vi "SDO_TRAJECTORY_EXECUTE_ABS.vi"(8 "Init":bool, 11 "End Pose ENG":T1={"TRANSLATION"={"X"=0.0, "Y"=0.0}, "ROTATION"={"VALUE"=0.0, "COS"=1.0, "SIN"=0.0}} {"ROTATION"."SIN" format="%13.4f"; "ROTATION"."COS" format="%13.4f"; "ROTATION"."VALUE" format="%13.4f"; "TRANSLATION"."Y" format="%14.3f"; "TRANSLATION"."X" format="%14.3f"}) -> (0 "AtReference":bool, 3 "Chassis Velocity Target":T4 {"vOmega" format="%10.3f"; "vY" format="%10.3f"; "vX" format="%10.3f"})   [LabVIEW 2023]
uses:
  <vilib>/Rock Robotics/WPI/ThirdParty/JAS_Junk/TrajLib/Trajectory_Library.lvlib
  SDO_TRAJECTORY_GLOBALS.vi
  <vilib>/Rock Robotics/WPI/ThirdParty/JAS_Junk/TrajLib/TypeDef/CHASSIS_SPEEDS.ctl
  <vilib>/Rock Robotics/WPI/ThirdParty/JAS_Junk/TrajLib/TypeDef/TRANSLATION2D.ctl
  <vilib>/Rock Robotics/WPI/ThirdParty/JAS_Junk/TrajLib/TypeDef/ROTATION2D.ctl
  <vilib>/Rock Robotics/WPI/ThirdParty/JAS_Junk/TrajLib/TypeDef/POSE2D.ctl
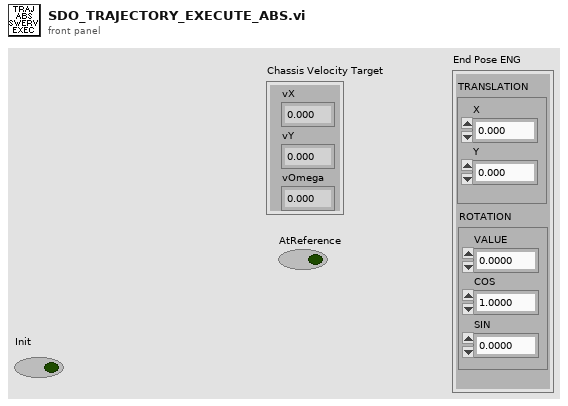
[diagram p1: front panel]
types:
  T1 = typedef "Trajectory_Library.lvlib/POSE2D.ctl" = cluster{"TRANSLATION":T2, "ROTATION":T3}
  T2 = typedef "Trajectory_Library.lvlib/TRANSLATION2D.ctl" = cluster{"X":dbl, "Y":dbl}
  T3 = typedef "Trajectory_Library.lvlib/ROTATION2D.ctl" = cluster{"VALUE":dbl, "COS":dbl, "SIN":dbl}
  T4 = typedef "Trajectory_Library.lvlib/CHASSIS_SPEEDS.ctl" = cluster{"vX":dbl, "vY":dbl, "vOmega":dbl}
  T5 = typedef "Trajectory_Library.lvlib/SWERVE_DRIVE_KINEMATICS.ctl" = cluster{"NumModules":i32, "InverseKinematics":T6, "ForwardKinematics":T6, "Modules":T2[], "PrevCoR":T2, "SavedModuleStates":T7[]}
  T6 = typedef "NI_Matrix.lvlib/RealMatrix.ctl" = dbl[][]
  T7 = typedef "Trajectory_Library.lvlib/SWERVE_DRIVE_MODULE_STATE.ctl" = cluster{"Speed":dbl, "Angle":T3}
  T8 = typedef "Trajectory_Library.lvlib/TRAJECTORY.ctl" = cluster{"TotalTImeSecs":dbl, "States":T9[]}
  T9 = typedef "Trajectory_Library.lvlib/TRAJ_STATE.ctl" = cluster{"TimeSeconds":dbl, "Velocity":dbl, "Acceleration":dbl, "POSE":T1, "Curvature":dbl}
  T10 = typedef "Trajectory_Library.lvlib/PID_TUNING.ctl" = cluster{"Kp":dbl, "Ki":dbl, "Kd":dbl, "MaximumIntegral":dbl, "MinimumIntegral":dbl}
  T11 = typedef "Trajectory_Library.lvlib/PROFILED_PID_CONTROLLER.ctl" = cluster{"Controller":T12, "Goal":T13, "Setpoint":T13, "Constraint":T14}
  T12 = typedef "Trajectory_Library.lvlib/PID_CONTROLLER.ctl" = cluster{"Kp":dbl, "Ki":dbl, "Kd":dbl, "Period":dbl, "Max_Integral":dbl, "Min_Integral":dbl, "Max_Input":dbl, "Min_Input":dbl, "Continuous":bool, "PositionError":dbl, "VelocityError":dbl, "PrevError":dbl, "TotalError":dbl, "PositionTolerance":dbl, "VelocityTolerance":dbl, "SetPoint":dbl, "Kf":dbl, "Prev_Deriv":dbl, "Prev_Deriv 2":dbl, "DerivativeFilter":bool, "Min_Output":dbl, "Max_Output":dbl, "Prev_F_P":dbl, "Prev_F_P_2":dbl, "AntiWindupActive":bool, "Measurement":dbl}
  T13 = typedef "Trajectory_Library.lvlib/TRAPEZOID_PROFILE_STATE.ctl" = cluster{"Position":dbl, "Velocity":dbl}
  T14 = typedef "Trajectory_Library.lvlib/TRAPEZOID_PROFILE_CONSTRAINT.ctl" = cluster{"MaxVelocity":dbl, "MaxAcceleration":dbl}
  T15 = typedef "Trajectory_Library.lvlib/HOLONOMIC_PACK_TUNING.ctl" = cluster{"X PID Tuning":T10, "Y PID Tuning":T10, "thetaProfiledPID_CTRL":T11}
  T16 = typedef "Trajectory_Library.lvlib/HOLONOMIC_DRV_CTRL.ctl" = cluster{"poseTolerance":T1, "poseError":T1, "Enabled":bool, "PID_xCtrl":T12, "PID_yCtrl":T12, "PROF_PID_thetaCtrl":T11, "RotationError":T3, "FirstRun":bool}
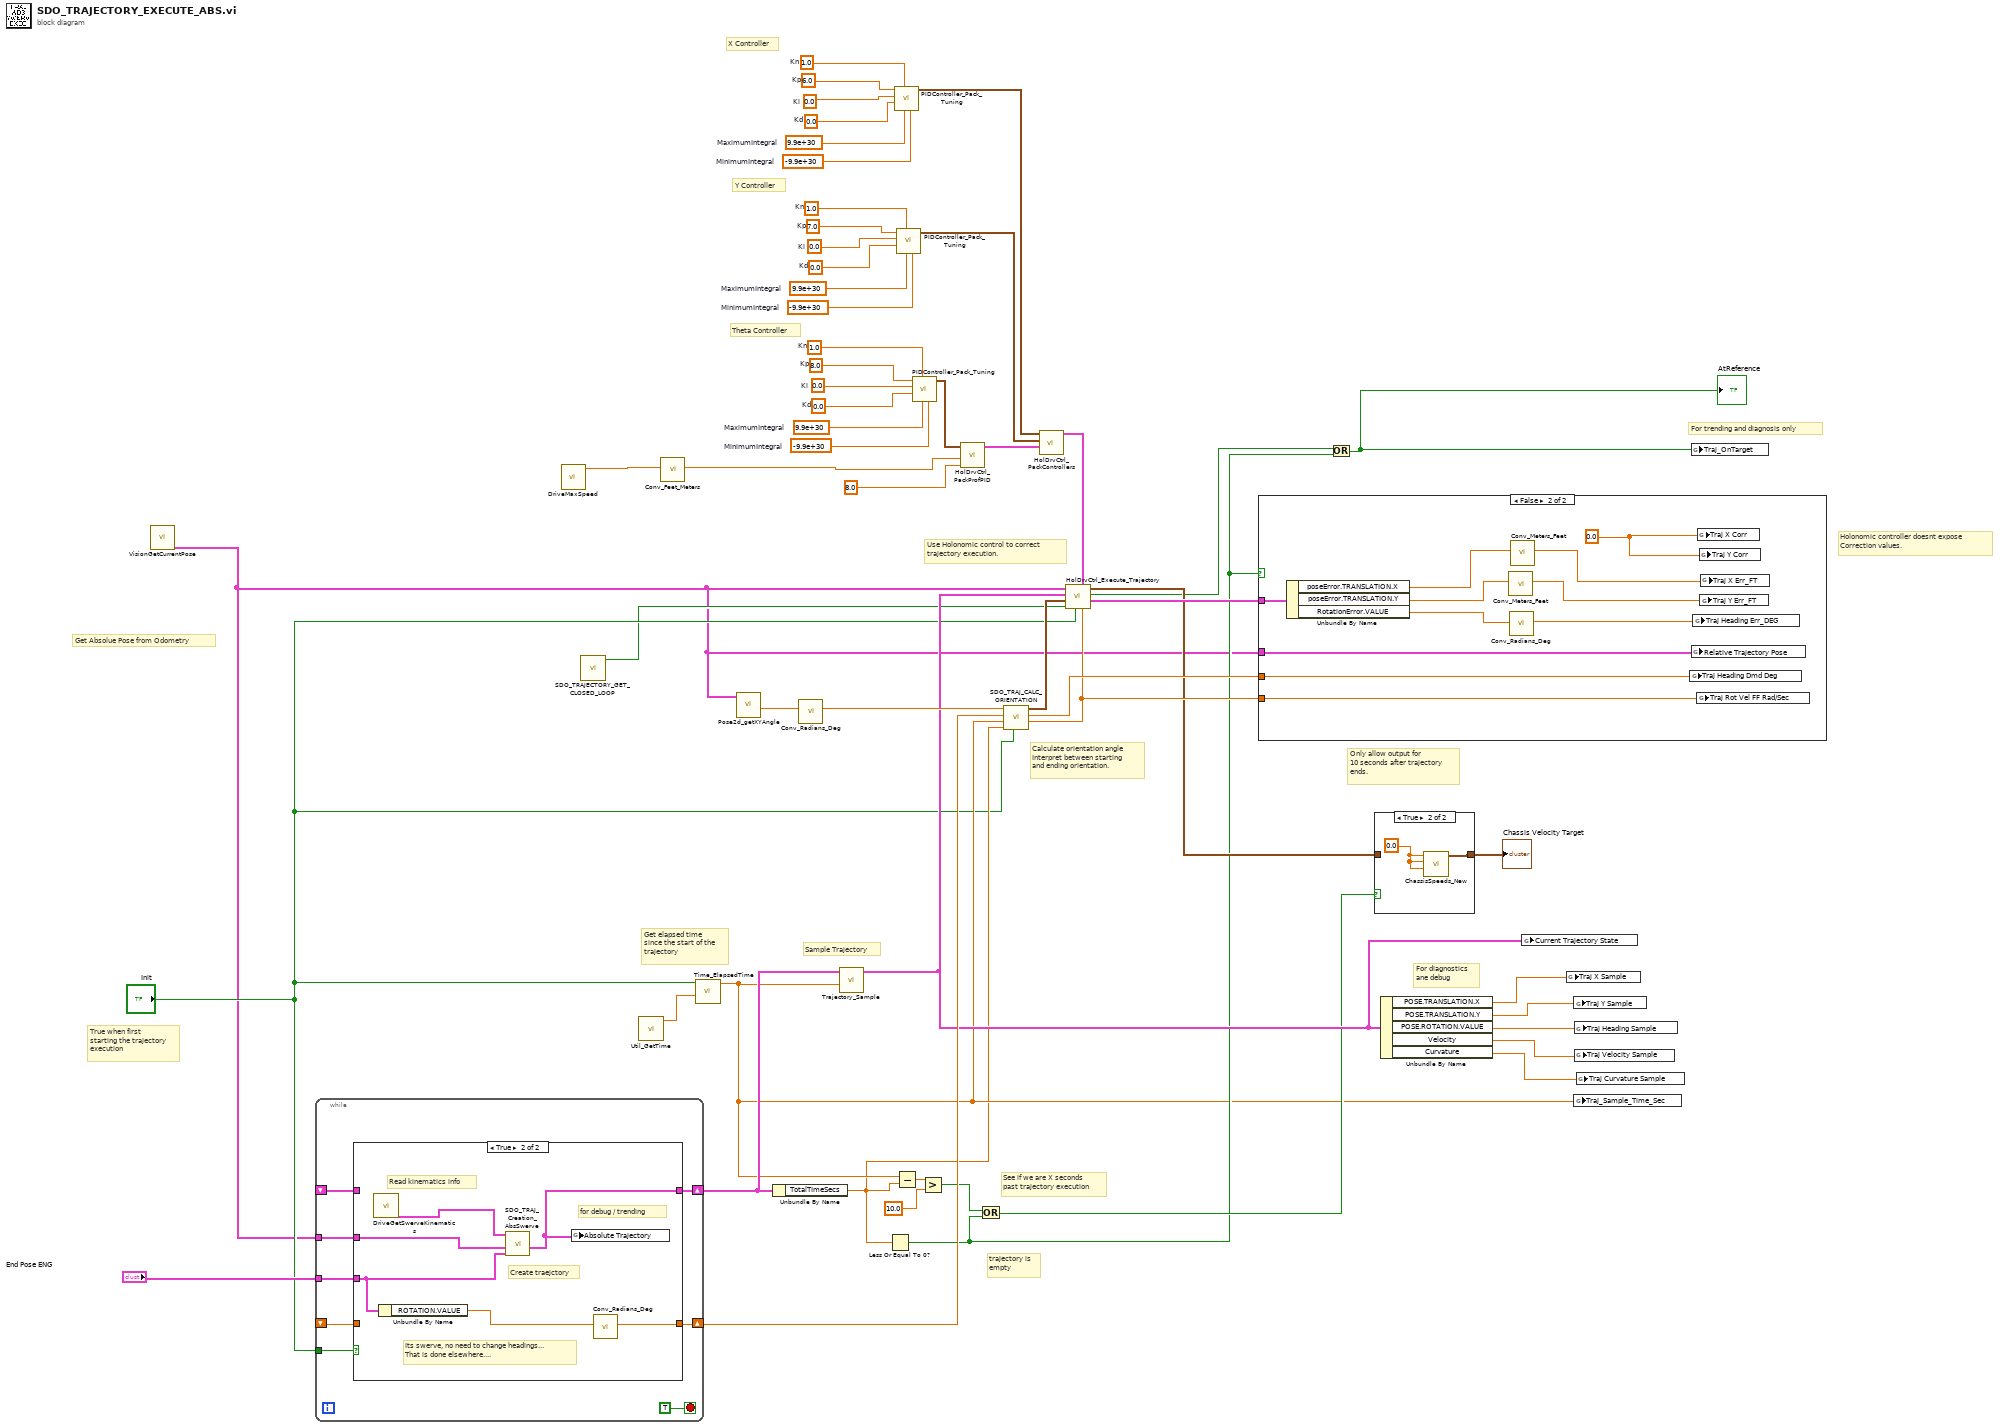
[diagram p0: block diagram]
diagram:
  w27 = 1.0  # Kn
  w30 = 8.0  # Kp
  w39 = 0.0  # Ki
  w40 = 0.0  # Kd
  w41 = 9.9e+30  # MaximumIntegral
  w42 = -9.9e+30  # MinimumIntegral
  w25 = 1.0  # Kn
  w28 = 6.0  # Kp
  w31 = 0.0  # Ki
  w32 = 0.0  # Kd
  w33 = 9.9e+30  # MaximumIntegral
  w34 = -9.9e+30  # MinimumIntegral
  w26 = 1.0  # Kn
  w29 = 7.0  # Kp
  w35 = 0.0  # Ki
  w36 = 0.0  # Kd
  w37 = 9.9e+30  # MaximumIntegral
  w38 = -9.9e+30  # MinimumIntegral
  # "trajectory is \nempty"
  # "Theta Controller"
  # "Y Controller"
  # "X Controller"
  # "Calculate orientation angle\nInterpret between starting\nand ending orientation."
  # "True when first\nstarting the trajectory\nexecution"
  # "Get elapsed time\nsince the start of the\ntrajectory"
  # "Holonomic controller doesnt expose\nCorrection values."
  # "Use Holonomic control to correct\ntrajectory execution."
  # "For trending and diagnosis only"
  # "For diagnostics\nane debug"
  # "Get Absolue Pose from Odometry"
  # "Sample Trajectory"
  # "See if we are X seconds \npast trajectory execution"
  # "Only allow output for\n10 seconds after trajectory\nends."
  n1 = call "VisionGetCurrentPose.vi"() -> ("Current Pose"=w1:T1)  [unwired: 9 in]
  n2 = while {
    tunnel: "Init" -> [w63]
    tunnel: w1 -> [w62]
    shift-right: [w61] -> w19
    shift-left: _ -> [w60]
    shift-right: [w59] -> w16
    shift-left: _ -> [w58]
    tunnel: "End Pose ENG" -> [w57]
    stop <- TRUE stop-if-true
    n3 = case shown="True" w63 {
      tunnel: w62 -> [_ w68]
      tunnel: [w66 w69] -> w61
      tunnel: w60 -> [w66 _]
      tunnel: [w65 w71] -> w59
      tunnel: w58 -> [w65 _]
      tunnel: w57 -> [_ w72]
      frame False {
      }
      frame True {
        # "for debug / trending"
        # "Read kinematics info"
        # "Its swerve, no need to change headings...\nThat is done elsewhere...."
        # "Create traejctory"
        n4 = call "DriveGetSwerveKinematics.vi"() -> ("SWERVE_DRIVE_KINEMATICS"=w67:T5)  [unwired: 11 in]
        n5 = Unbundle By Name(w72) -> ("ROTATION.VALUE"=w70:dbl)
        n6 = call "SDO_TRAJ_Creation_AbsSwerve.vi"("End Pose  ENG"=w72, "Current Pose SI"=w68, "SWERVE_DRIVE_KINEMATICS"=w67) -> ("Absolute Trajectory"=w69:T8)  [unwired: 6 in, 2 out]
        n7 = global write "SDO_TRAJECTORY_GLOBALS.vi" "Absolute Trajectory"(w69) -> ()
        n8 = call <vilib>:"Conv_Radians_Deg.vi"("Radians"=w70) -> ("Degrees"=w71:dbl)  [unwired: 10 in]
      }
    }
  }
  n9 = call "DriveMaxSpeed.vi"() -> ("Max Speed (ft/sec)"=w3:dbl)  [unwired: 11 in]
  n10 = call "SDO_TRAJECTORY_GET_CLOSED_LOOP.vi"() -> ("AUTO_CLOSED_LOOP"=w4:bool)  [unwired: 11 in]
  n11 = call <vilib>:"Util_GetTime.vi"() -> ("FPGA_Time_Seconds"=w53:dbl)  [unwired: 9 in, 2 out]
  n12 = call <vilib>:"Conv_Feet_Meters.vi"("Feet"=w3) -> ("Meters"=w2:dbl)  [unwired: 10 in]
  n13 = call <vilib>:"Time_ElapsedTime.vi"("PassthroughTime_SEC"=w53, "Reset"="Init") -> ("Elapsed Time Sec"=w7:dbl)  [unwired: 9 in]
  n14 = call <vilib>:"Pose2d_getXYAngle.vi"("in POSE"=w1) -> ("Angle"=w18:dbl)  [unwired: 8 in, 2 out]
  n15 = Unbundle By Name(w19) -> ("TotalTImeSecs"=w6:dbl)
  n16 = call <vilib>:"Conv_Radians_Deg.vi"("Radians"=w18) -> ("Degrees"=w17:dbl)  [unwired: 10 in]
  n17 = call <vilib>:"Trajectory_Sample.vi"("Time"=w7, "InputTRAJECTORY"=w19) -> ("OutputTRAJ_STATE"=w15:T9)  [unwired: 9 in]
  n18 = Less Or Equal To 0?(x=w6) -> (x <= 0?=w8:bool)
  n19 = call <vilib>:"PIDController_Pack_Tuning.vi"("MinimumIntegral"=w34, "MaximumIntegral"=w33, "Kn"=w25, "Kd"=w32, "Ki"=w31, "Kp"=w28) -> ("PID Tuning"=w43:T10)  [unwired: 5 in]
  n20 = Subtract(x=w7, y=w6) -> (x-y=w56:dbl)
  n21 = call <vilib>:"PIDController_Pack_Tuning.vi"("MinimumIntegral"=w38, "MaximumIntegral"=w37, "Kn"=w26, "Kd"=w36, "Ki"=w35, "Kp"=w29) -> ("PID Tuning"=w44:T10)  [unwired: 5 in]
  n22 = call <vilib>:"PIDController_Pack_Tuning.vi"("MinimumIntegral"=w42, "MaximumIntegral"=w41, "Kn"=w27, "Kd"=w40, "Ki"=w39, "Kp"=w30) -> ("PID Tuning"=w24:T10)  [unwired: 5 in]
  n23 = Greater?(x=w56, y=10.0) -> (0:w12:bool)
  n24 = call <vilib>:"HolDrvCtrl_PackProfPID.vi"("Max Accel"=8.0, "Max Speed"=w2, "Theta PID Tuning"=w24) -> ("Theta PID CONTROLLER"=w45:T11)  [unwired: 8 in]
  n25 = Or(x=w12, y=w8) -> (x .or. y?=w11:bool)
  n26 = call "SDO_TRAJ_CALC_ORIENTATION.vi"("Init"="Init", "Total Trajectory Time Sec"=w6, "Elapsed Traj Time Sec"=w7, "End Orientation Demand DEG"=w16, "Starting Orientation  DEG"=w17) -> ("Rotational Velocity Rad Per Sec"=w21:dbl, "Orientation Demand Deg"=w47:dbl, "Orientation Demand"=w23:T3)  [unwired: 4 in]
  n27 = call <vilib>:"HolDrvCtrl_PackControllers.vi"("thetaProfiledPID_CTRL"=w45, "Y PID Tuning"=w44, "X PID Tuning"=w43) -> ("HOLONOMIC_CTRL_PACK_TUNING"=w46:T15)  [unwired: 8 in]
  n28 = call <vilib>:"HolDrvCtrl_Execute_Trajectory.vi"("Rotational Velocity Feedforward \nRad/Sec"=w21, "HOLONOMIC_CTRL_PACK_TUNING"=w46, "Reset"="Init", "Enable"=w4, "angleRef"=w23, "desiredTrajState"=w15, "currentPose"=w1) -> ("outHOLONOMIC_DRV_CTRL"=w22:T16, "AtReference"=w10:bool, "calcChassisSpeed"=w13:T4)  [unwired: 2 in]
  n29 = case shown="False" w8 {
    tunnel: w47 -> [_ w82]
    tunnel: w22 -> [_ w76]
    tunnel: w21 -> [_ w75]
    tunnel: w1 -> [_ w73]
    frame True {
    }
    frame False {
      w83 = 0.0 ("Y Corr")
      n30 = Unbundle By Name(w76) -> ("poseError.TRANSLATION.X"=w80:dbl, "poseError.TRANSLATION.Y"=w79:dbl, "RotationError.VALUE"=w74:dbl)
      n31 = call <vilib>:"Conv_Meters_Feet.vi"("Meters"=w79) -> ("Feet"=w78:dbl)  [unwired: 10 in]
      n32 = call <vilib>:"Conv_Radians_Deg.vi"("Radians"=w74) -> ("Degrees"=w81:dbl)  [unwired: 10 in]
      n33 = call <vilib>:"Conv_Meters_Feet.vi"("Meters"=w80) -> ("Feet"=w77:dbl)  [unwired: 10 in]
      n34 = global write "SDO_TRAJECTORY_GLOBALS.vi" "Traj Heading Dmd Deg"(w82) -> ()
      n35 = global write "SDO_TRAJECTORY_GLOBALS.vi" "Relative Trajectory Pose"(w73) -> ()
      n36 = global write "SDO_TRAJECTORY_GLOBALS.vi" "Traj Heading Err_DEG"(w81) -> ()
      n37 = global write "SDO_TRAJECTORY_GLOBALS.vi" "Traj Rot Vel FF Rad/Sec"(w75) -> ()
      n38 = global write "SDO_TRAJECTORY_GLOBALS.vi" "Traj X Corr"(w83) -> ()
      n39 = global write "SDO_TRAJECTORY_GLOBALS.vi" "Traj Y Corr"(w83) -> ()
      n40 = global write "SDO_TRAJECTORY_GLOBALS.vi" "Traj Y Err_FT"(w78) -> ()
      n41 = global write "SDO_TRAJECTORY_GLOBALS.vi" "Traj X Err_FT"(w77) -> ()
    }
  }
  n42 = Or(x=w10, y=w8) -> (x .or. y?=w9:bool)
  "AtReference" <- w9
  n43 = case shown="True" w11 {
    tunnel: w13 -> [w84 _]
    tunnel: [w84 w85] -> w54
    frame False {
    }
    frame True {
      w86 = 0.0 ("vX")
      n44 = call <vilib>:"ChassisSpeeds_New.vi"("vAngular"=w86, "vY"=w86, "vX"=w86) -> ("CHASSIS"=w85:T4)  [unwired: 8 in]
    }
  }
  "Chassis Velocity Target" <- w54
  n45 = Unbundle By Name(w15) -> ("POSE.TRANSLATION.X"=w52:dbl, "POSE.TRANSLATION.Y"=w51:dbl, "POSE.ROTATION.VALUE"=w50:dbl, "Velocity"=w49:dbl, "Curvature"=w48:dbl)
  n46 = global write "SDO_TRAJECTORY_GLOBALS.vi" "Current Trajectory State"(w15) -> ()
  n47 = global write "SDO_TRAJECTORY_GLOBALS.vi" "Traj X Sample"(w52) -> ()
  n48 = global write "SDO_TRAJECTORY_GLOBALS.vi" "Traj Y Sample"(w51) -> ()
  n49 = global write "SDO_TRAJECTORY_GLOBALS.vi" "Traj_Sample_Time_Sec"(w7) -> ()
  n50 = global write "SDO_TRAJECTORY_GLOBALS.vi" "Traj Heading Sample"(w50) -> ()
  n51 = global write "SDO_TRAJECTORY_GLOBALS.vi" "Traj Velocity Sample"(w49) -> ()
  n52 = global write "SDO_TRAJECTORY_GLOBALS.vi" "Traj Curvature Sample"(w48) -> ()
  n53 = global write "SDO_TRAJECTORY_GLOBALS.vi" "Traj_OnTarget"(w9) -> ()
